vi "UserDecoder.vi"(0 "input bit stream":i8[](array[numeric]), 1 "Sync length":i32, 2 "Refnum in":T1, 5 "RS n":i32, 7 "RS k":i32, 9 "Const. length":i32, 11 "error in (no error)":errorcluster, 13 "Tab Control in":enum32{"No coding", "RS only", "RS+Conv."}(ring)) -> (4 "output bit stream":i8[](array[numeric]), 8 "Refnum out":T1, 15 "error out":errorcluster)   [LabVIEW 2012]
uses:
  <vilib>/addons/Modulation/Digital/Support/Controls/MT Generic Refnum.ctl
  <vilib>/addons/Modulation/Digital/Channel Coding/MT RS Symbol Decoder (normal).vi
  <vilib>/addons/Modulation/Digital/Channel Coding/MT Convolutional Decoder (Viterbi Hard Decision, Rate).vi
  <vilib>/addons/Modulation/niDMT.lvlib
panel:
  out "Rx length 2":i32
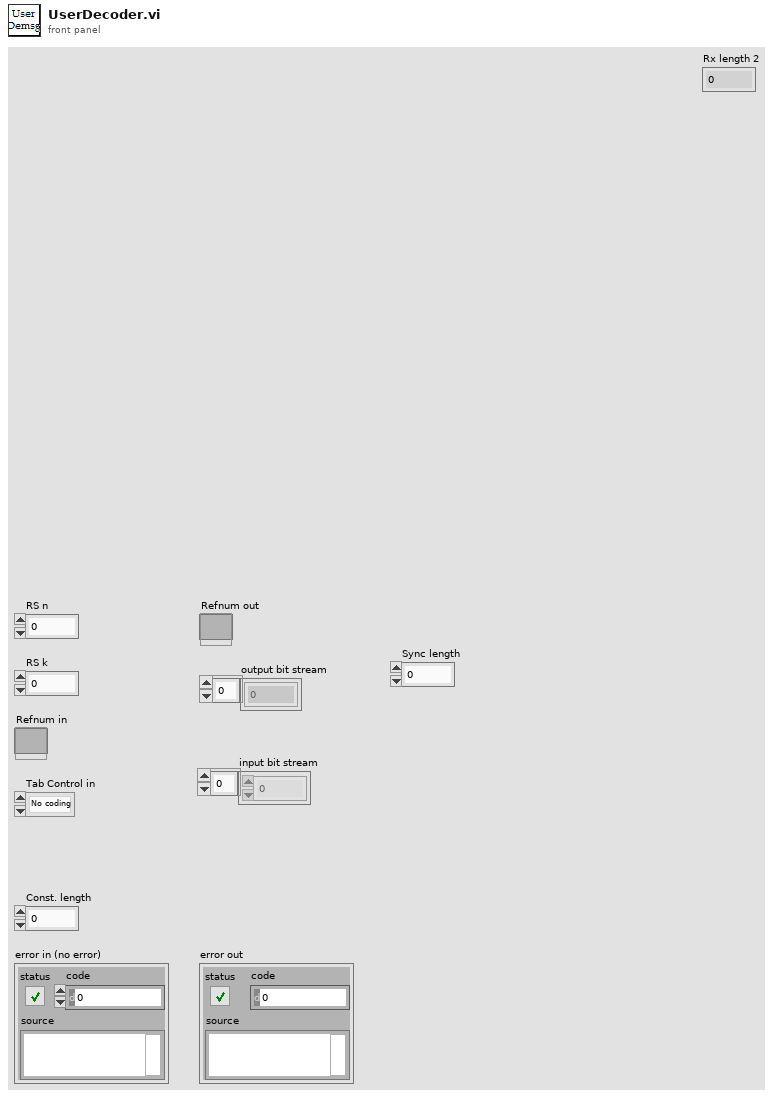
[diagram p1: front panel]
types:
  T1 = typedef "niDMT.lvlib/MT Generic Refnum.ctl" = refnum<k20>
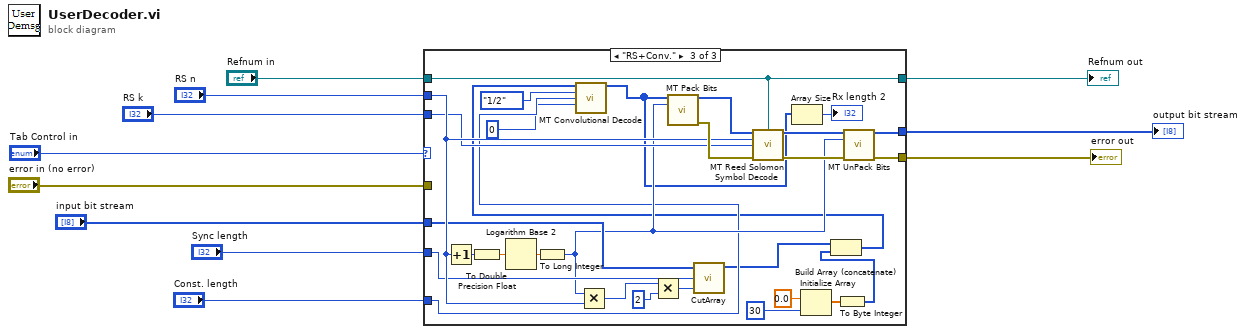
[diagram p0: block diagram]
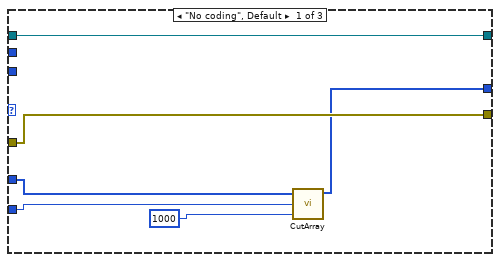
[diagram p2: hidden frame]
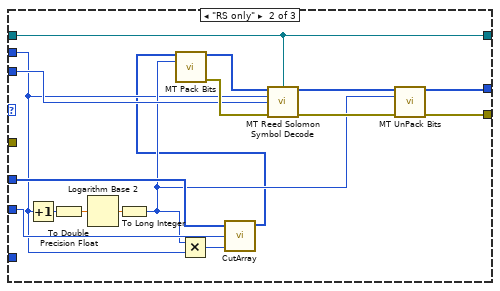
[diagram p3: hidden frame]
diagram:
  n1 = case shown="\"RS+Conv.\"" "Tab Control in" {
    tunnel: [w12 w31 w55] -> w4
    tunnel: "RS n" -> [_ w20 w56]
    tunnel: "RS k" -> [_ w24 w52]
    tunnel: "error in (no error)" -> [w16 _ _]
    tunnel: "Refnum in" -> [w17 w27 w53]
    tunnel: "Const. length" -> [_ _ w44]
    tunnel: [w17 w27 w53] -> w10
    tunnel: [w16 w30 w54] -> w11
    tunnel: "input bit stream" -> [w13 w23 w50]
    tunnel: "Sync length" -> [w14 w22 w51]
    frame "No coding", Default {
      n2 = call "CutArray.vi"("array"=w13, "From index"=w14, "Length"=1000 ("bits per integer")) -> ("Sub array"=w12:i8[])  [unwired: 5 in]
    }
    frame "RS only" {
      n3 = Increment(x=w20) -> (x+1=w33:i32)
      n4 = To Double Precision Float(number=w33) -> (double precision float=w34:dbl)
      n5 = Logarithm Base 2(1:w34) -> (0:w32:dbl)
      n6 = To Long Integer(number=w32) -> (32bit integer=w21:i32)
      n7 = Multiply(x=w21, y=w20) -> (x*y=w19:i32)
      n8 = call "CutArray.vi"("array"=w23, "From index"=w22, "Length"=w19) -> ("Sub array"=w18:i8[])  [unwired: 5 in]
      n9 = call <vilib>:"MT Pack Bits.vi"("input bit stream"=w18, "bits per integer"=w21) -> ("output integers"=w26:i32[], "error out"=w25:errorcluster)  [unwired: 12 in]
      n10 = call-poly <vilib>:"MT Reed Solomon Symbol Decode.vi"("input symbols"=w26, "modulation session"=w27, "code word length (n), symbols"=w20, "data word length (k), symbols"=w24, "error in (no error)"=w25) -> ("output symbols"=w28:i32[], "error out"=w29:errorcluster)  [unwired: 9 in]
      n11 = call <vilib>:"MT UnPack Bits.vi"("input integers"=w28, "bits per integer"=w21, "error in (no error)"=w29) -> ("output bit stream"=w31:i8[], "error out"=w30:errorcluster)  [unwired: 11 in]
    }
    frame "RS+Conv." {
      n12 = Increment(x=w56) -> (x+1=w58:i32)
      n13 = To Double Precision Float(number=w58) -> (double precision float=w57:dbl)
      n14 = Logarithm Base 2(1:w57) -> (0:w59:dbl)
      n15 = To Long Integer(number=w59) -> (32bit integer=w46:i32)
      n16 = Multiply(x=w46, y=w56) -> (x*y=w48:i32)
      n17 = Multiply(x=w48, y=2) -> (x*y=w49:i32)
      n18 = call "CutArray.vi"("array"=w50, "From index"=w51, "Length"=w49) -> ("Sub array"=w36:i8[])  [unwired: 5 in]
      n19 = Initialize Array(0.0 ("element"), 30 ("dimension size")) -> (w38:dbl[])
      n20 = To Byte Integer(number=w38) -> (8bit integer=w37:i8[])
      n21 = Build Array (concatenate)(w36, w37) -> (w35:i8[])
      n22 = call-poly <vilib>:"MT Convolutional Decode.vi"("input bit stream"=w35, "rate (k/n)"=enum16{"1/2", "1/3", "1/4", "2/3", "3/4"}."1/2", "constraint length (K)"=w44, "initial state"=u32 0) -> ("output bit stream"=w41:i8[])  [unwired: 9 in, 2 out]
      n23 = call <vilib>:"MT Pack Bits.vi"("input bit stream"=w41, "bits per integer"=w46) -> ("output integers"=w62:i32[], "error out"=w63:errorcluster)  [unwired: 12 in]
      n24 = call-poly <vilib>:"MT Reed Solomon Symbol Decode.vi"("input symbols"=w62, "modulation session"=w53, "code word length (n), symbols"=w56, "data word length (k), symbols"=w52, "error in (no error)"=w63) -> ("output symbols"=w61:i32[], "error out"=w60:errorcluster)  [unwired: 9 in]
      n25 = Array Size(array=w41) -> (size(s)=→"Rx length 2":i32)
      n26 = call <vilib>:"MT UnPack Bits.vi"("input integers"=w61, "bits per integer"=w46, "error in (no error)"=w60) -> ("output bit stream"=w55:i8[], "error out"=w54:errorcluster)  [unwired: 11 in]
    }
  }
  "error out" <- w11
  "Refnum out" <- w10
  "output bit stream" <- w4
